vi "GMM.vi"(0 "Array":dbl[][](array[numeric])) -> (1 "Group 1":dbl, 2 "Group 2":dbl)   [LabVIEW 2013]
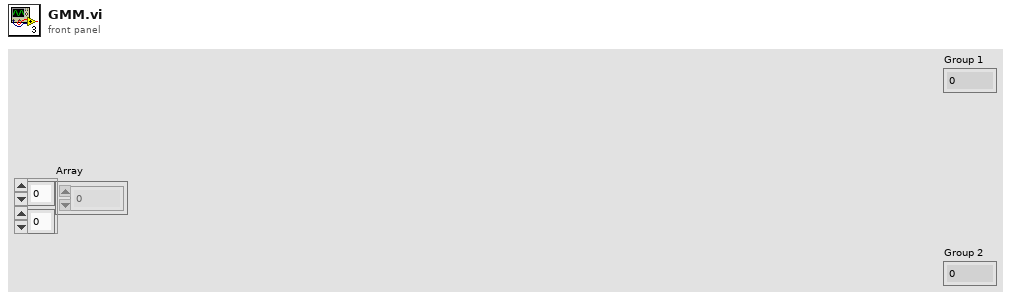
[diagram p1: front panel]
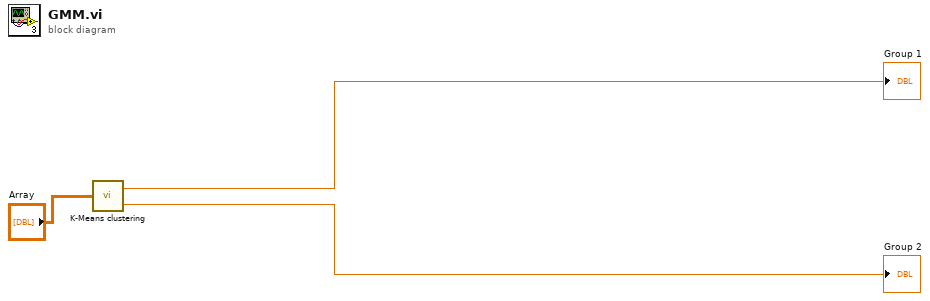
[diagram p0: block diagram]
diagram:
  n1 = call "K-Means clustering.vi"("Array"="Array") -> ("Mean 1"=→"Group 1":dbl, "Mean 2"=→"Group 2":dbl)
